vi "Find FPGA Addon.vi"(8 "error in":errorcluster, 10 "FPGA addon name":string, 11 "target in":refnum<k39>) -> (0 "error out":errorcluster, 1 "found ?":bool, 2 "FPGA addon refnum out":T1=18446744073709551615 format="%.0x", 3 "target out":refnum<k39>)   [LabVIEW 2026, in "Scripting API.lvlib"]
doc: "Checks if an FPGA addon custom device, with the provided name exists within the specified system definition target. If an FPGA addon custom device exists, this VI will return it's reference."
uses:
  Scripting API.lvlib
  C:/Users/Administrator/Desktop/Jatin/All DNC DLLs/NationalInstruments.VeriStand.SystemDefinitionAPI.dll
  Jatin/All DNC DLLs/NationalInstruments.VeriStand.SystemDefinitionAPI.dll
  <vilib>/NI VeriStand/Custom Device API/Custom Device Item Ref.ctl
  Addon/Addon Shared/SubVIs/Constants.vi
  <vilib>/NI VeriStand/Custom Device API/Custom Device API.lvlib
  Addon/Addon Shared/FPGA Addon Shared.lvlib
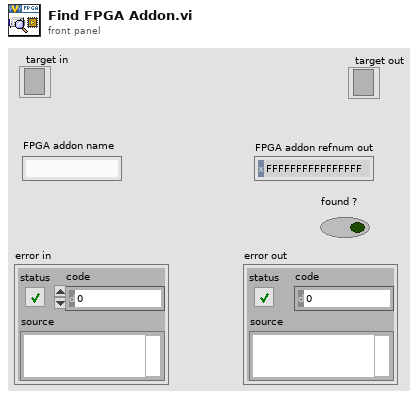
[diagram p1: front panel]
types:
  T1 = typedef "Custom Device API.lvlib/Custom Device Item Ref.ctl" = u64
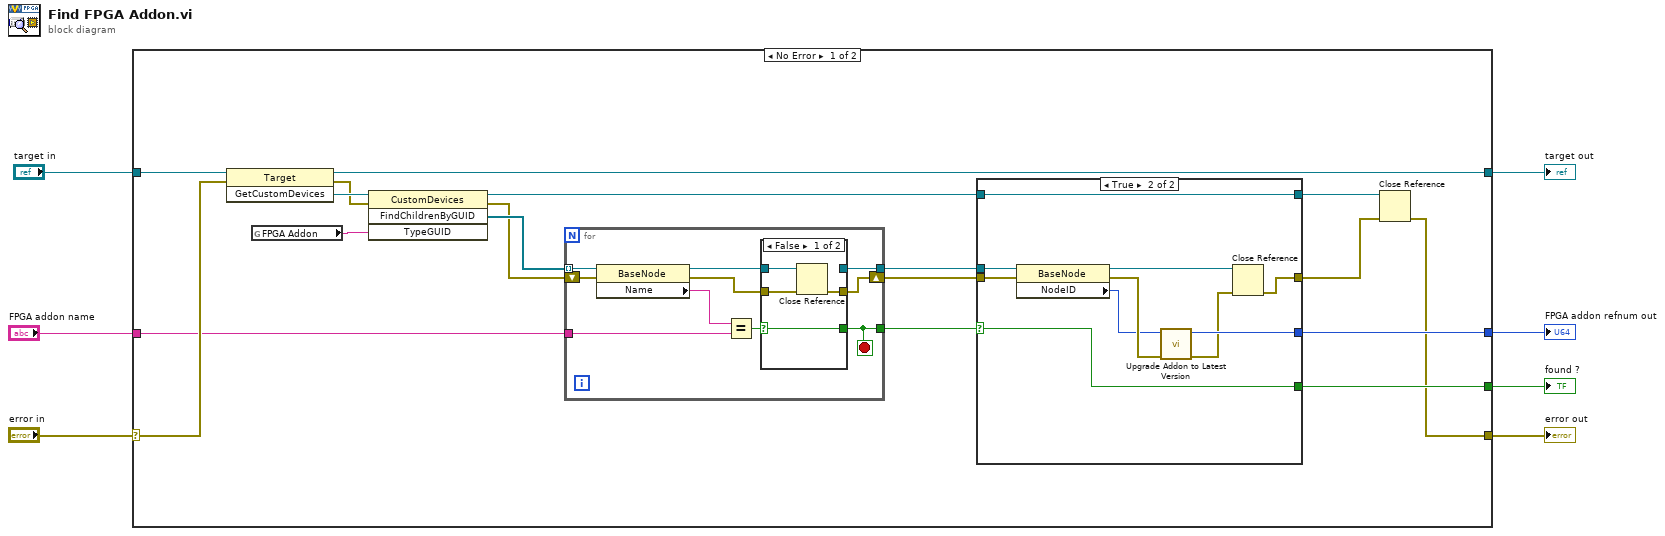
[diagram p0: block diagram]
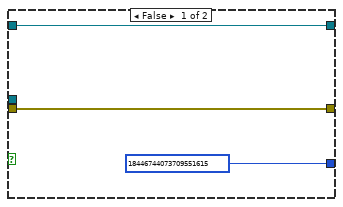
[diagram p3: hidden frame]
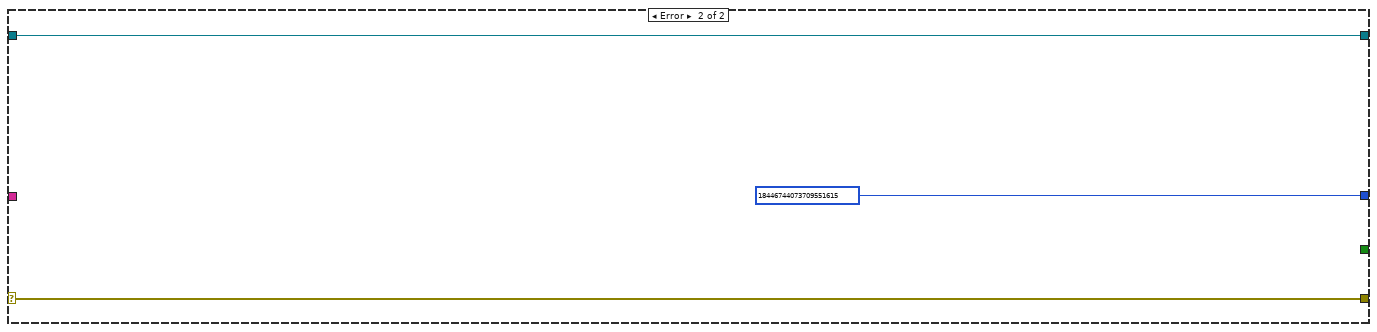
[diagram p4: hidden frame]
diagram:
  n1 = case shown="No Error" "error in" {
    selector: "error in" -> [w24 w58]
    tunnel: [w25 w56] -> w1
    tunnel: [w20 w58] -> w4
    tunnel: "target in" -> [w23 w56]
    tunnel: "FPGA addon name" -> [w16 _]
    tunnel: [w22 T1 18446744073709551615 ("FPGA Addon refnum")] -> w3
    tunnel: [w21 _] -> w2
    frame No Error {
      n2 = invoke class="Target" method="GetCustomDevices"(reference=w23, error in=w24) -> (reference out=w25:refnum<k39>, error out=w15:errorcluster, "GetCustomDevices"=w17:refnum<k39>)  [unwired: 1 in]
      n3 = global read "Constants.vi" "FPGA Addon"() -> (w18:string)
      n4 = invoke class="CustomDevices" method="FindChildrenByGUID"(reference=w17, error in=w15, "TypeGUID"=w18) -> (reference out=w11:refnum<k39>, error out=w14:errorcluster, "FindChildrenByGUID"=w19:refnum<k39>[])  [unwired: 1 in, 1 out]
      n5 = for {
        tunnel: w19 -> [w35] mode=indexing
        tunnel: w16 -> [w33]
        shift-right: [w28] -> w8
        shift-left: w14 -> [w31]
        tunnel: [w27] -> w13
        tunnel: [w26] -> w12
        stop <- w26 stop-if-true
        n6 = property class="BaseNode"(reference=w35, error in=w31) -> (reference out=w30:refnum<k39>, error out=w29:errorcluster, "Name"=w34:string)
        n7 = Equal?(x=w34, y=w33) -> (x = y?=w32:bool)
        n8 = case shown="False" w32 {
          selector: w32 -> [w36 w40]
          tunnel: w30 -> [w39 w42]
          tunnel: w29 -> [w38 w41]
          tunnel: [w37 w41] -> w28
          tunnel: [_ w42] -> w27
          tunnel: [w36 w40] -> w26
          frame False {
            n9 = Close Reference(reference=w39, error in (no error)=w38) -> (error out=w37:errorcluster)
          }
          frame True {
          }
        }
      }
      n10 = case shown="True" w12 {
        selector: w12 -> [_ w50]
        tunnel: [T1 18446744073709551615 ("FPGA Addon refnum") w47] -> w22
        tunnel: [_ w50] -> w21
        tunnel: w13 -> [_ w55]
        tunnel: w11 -> [w44 w54]
        tunnel: [w44 w54] -> w10
        tunnel: [w43 w52] -> w9
        tunnel: w8 -> [w43 w51]
        frame False {
        }
        frame True {
          n11 = property class="BaseNode"(reference=w55, error in=w51) -> (reference out=w53:refnum<k39>, error out=w49:errorcluster, "NodeID"=w48:u64)
          n12 = call "Upgrade Addon to Latest Version.vi"("error in (no error)"=w49, "Device Item Ref in in"=w48) -> ("error out"=w46:errorcluster, "Device Item Ref out"=w47:T1)  [unwired: 8 in]
          n13 = Close Reference(reference=w53, error in (no error)=w46) -> (error out=w52:errorcluster)
        }
      }
      n14 = Close Reference(reference=w10, error in (no error)=w9) -> (error out=w20:errorcluster)
    }
    frame Error {
    }
  }
  "target out" <- w1
  "error out" <- w4
  "FPGA addon refnum out" <- w3
  "found ?" <- w2
